vi "set last calibration.vi"(8 "error in (no error)":errorcluster caption="Fehler (Eingang, kein Fehler)", 10 "last calibration":string, 11 "Device (Eingang)":refnum<class "Device.lvclass">) -> (0 "error out":errorcluster caption="Fehler (Ausgang)", 3 "Device (Ausgang)":refnum<class "Device.lvclass">)   [LabVIEW 2013, in "DatenKlassen.lvlib" / "Device.lvclass"]
uses:
  Device.lvclass
  Device.lvclass/Device.ctl
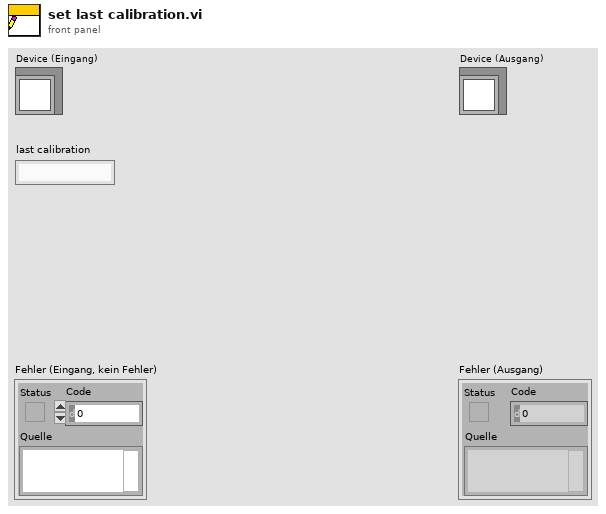
[diagram p1: front panel]
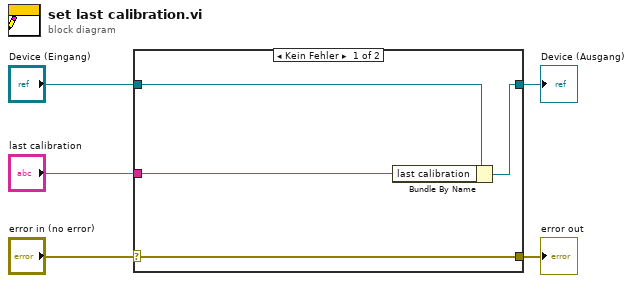
[diagram p0: block diagram]
diagram:
  n1 = case shown="Kein Fehler" "error in (no error)" {
    selector: "error in (no error)" -> [w9 w10]
    tunnel: [w9 w10] -> w4
    tunnel: [w7 w11] -> w2
    tunnel: "Device (Eingang)" -> [w8 w11]
    tunnel: "last calibration" -> [w6 _]
    frame No Error {
      n2 = Bundle By Name(cluster=w8, "last calibration"=w6) -> (w7:refnum<class "Device.lvclass">)
    }
    frame Error {
    }
  }
  "error out" <- w4
  "Device (Ausgang)" <- w2
